vi "createPlayer.vi"(8 "error in (no error)":errorcluster) -> (0 "error out":errorcluster, 3 "Player out":refnum<class "Player.lvclass">)   [LabVIEW 2019, in "Player.lvclass"]
uses:
  Player.lvclass
  Player.lvclass/Player.ctl
panel:
  in  "Name":string
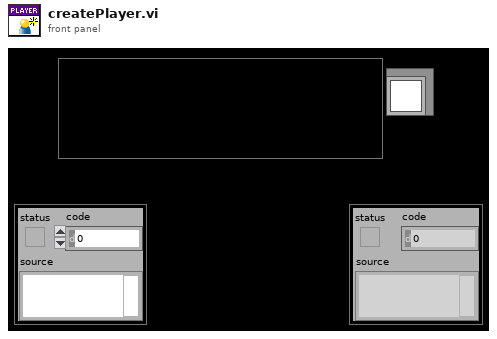
[diagram p1: front panel]
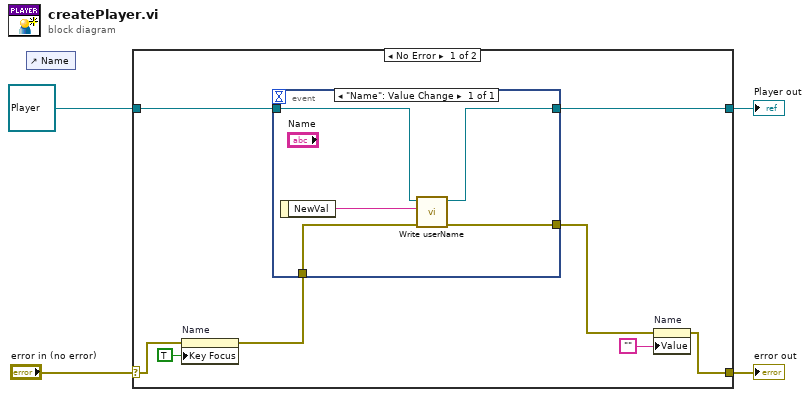
[diagram p0: block diagram]
diagram:
  n1 = control-ref of="Name"() -> ()  [unwired: 1 out]
  n2 = case shown="No Error" "error in (no error)" {
    selector: "error in (no error)" -> [w6 w19]
    tunnel: [w9 w19] -> w3
    tunnel: [w11 w18] -> w1
    tunnel: refnum<class "Player.lvclass"> refnum ("Player in") -> [w12 w18]
    frame No Error {
      n3 = property on="Name" class="Str"(error in=w6, "Key Focus"=TRUE) -> (error out=w5:errorcluster)  [unwired: 1 in, 1 out]
      n4 = event shown="[0] \"Name\": Value Change" {
        selector: _ -> [_]
        dyn-events: _ -> [_]
        timeout: _ -> [_]
        tunnel: w5 -> [w17]
        tunnel: [w16] -> w10
        tunnel: w12 -> [w15]
        tunnel: [w14] -> w11
        event "Name": Value Change {
          n5 = event-data() -> ("NewVal"=w13:string)  [unwired: 1 in]
          n6 = call "Write userName.vi"("error in (no error)"=w17, "userName"=w13, "Player in"=w15) -> ("error out"=w16:errorcluster, "Player out"=w14:refnum<class "Player.lvclass">)  [unwired: 7 in]
        }
      }
      n7 = property on="Name" class="Str"(error in=w10, "Value"="") -> (error out=w9:errorcluster)  [unwired: 1 in, 1 out]
    }
    frame Error {
    }
  }
  "error out" <- w3
  "Player out" <- w1
